vi "EditorThumbnail init.vi"(8 "error in (no error)":errorcluster, 11 "EditThumbnail in":refnum<class "EditorThumbnail.lvclass">) -> (0 "error out":errorcluster, 3 "EditThumbnail out":refnum<class "EditorThumbnail.lvclass">)   [LabVIEW 2018, in "EditorThumbnail.lvclass"]
uses:
  EditorThumbnail.lvclass
  EditorThumbnail.lvclass/EditorThumbnail.ctl
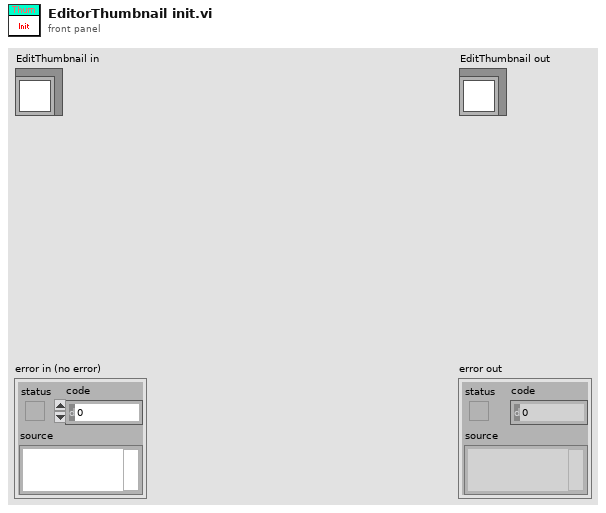
[diagram p1: front panel]
types:
  T1 = cluster{"index":u32, "data":cluster{"xdata":dbl[], "ydata":sgl[]}[], "peak":dbl[], "picture":picture}[]
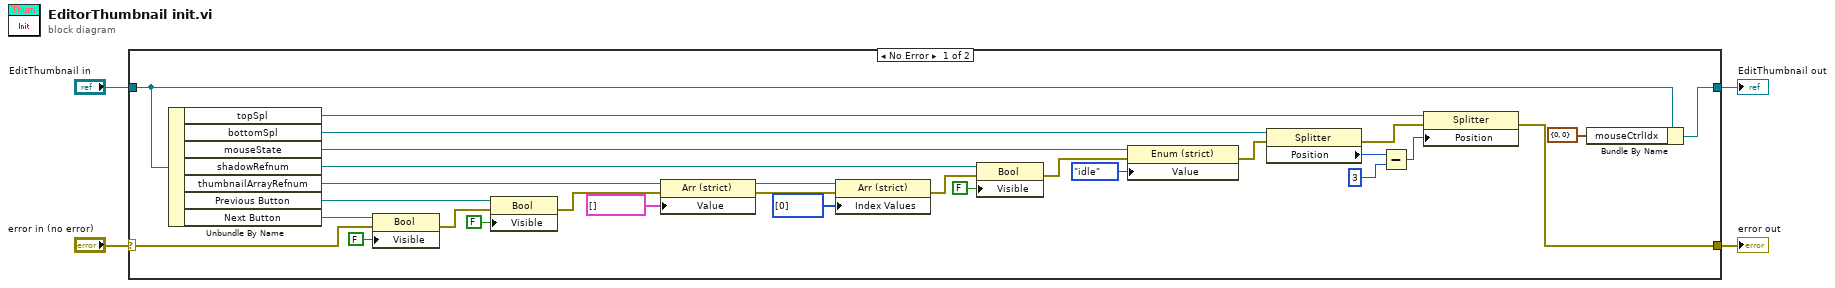
[diagram p0: block diagram]
diagram:
  n1 = case shown="No Error" "error in (no error)" {
    selector: "error in (no error)" -> [w13 w35]
    tunnel: [w8 w35] -> w3
    tunnel: [w21 w34] -> w1
    tunnel: "EditThumbnail in" -> [w23 w34]
    frame No Error {
      n2 = Unbundle By Name(w23) -> ("topSpl"=w10:refnum<vi>, "bottomSpl"=w12:refnum<vi>, "mouseState"=w26:refnum<vi>, "shadowRefnum"=w30:refnum<vi>, "thumbnailArrayRefnum"=w20:refnum<vi>, "Previous Button"=w18:refnum<vi>, "Next Button"=w19:refnum<vi>)
      n3 = property class="Bool"(reference=w19, error in=w13, "Visible"=FALSE) -> (error out=w17:errorcluster)  [unwired: 1 out]
      n4 = property class="Bool"(reference=w18, error in=w17, "Visible"=FALSE) -> (error out=w14:errorcluster)  [unwired: 1 out]
      n5 = property class="Arr (strict)"(reference=w20, error in=w14, "Value"=T1 []) -> (reference out=w33:refnum<vi>, error out=w32:errorcluster)
      n6 = property class="Arr (strict)"(reference=w33, error in=w32, "Index Values"=u32[] [0]) -> (error out=w28:errorcluster)  [unwired: 1 out]
      n7 = property class="Bool"(reference=w30, error in=w28, "Visible"=FALSE) -> (error out=w24:errorcluster)  [unwired: 1 out]
      n8 = property class="Enum (strict)"(reference=w26, error in=w24, "Value"=enum16{"idle", "down", "move", "up"}."idle") -> (error out=w11:errorcluster)  [unwired: 1 out]
      n9 = property class="Splitter"(reference=w12, error in=w11) -> (error out=w9:errorcluster, "Position"=w7:i32)  [unwired: 1 out]
      n10 = Subtract(x=w7, y=3) -> (x-y=w5:i32)
      n11 = property class="Splitter"(reference=w10, error in=w9, "Position"=w5) -> (error out=w8:errorcluster)  [unwired: 1 out]
      n12 = Bundle By Name(cluster=w23, "mouseCtrlIdx"=cluster{"downIdx":i32, "upIdx":i32} {"downIdx"=0, "upIdx"=0}) -> (w21:refnum<class "EditorThumbnail.lvclass">)
    }
    frame Error {
    }
  }
  "error out" <- w3
  "EditThumbnail out" <- w1
